vi "jitterPlot.vi"(8 "Y-jitter":dbl=0.03, 9 "X-jitter":dbl=0.03, 11 "PlotCluster":cluster{"X":dbl[], "Y":dbl[]}) -> (3 "JitteredPlotCluster":cluster{"X":dbl[], "Y":dbl[]})   [LabVIEW 2013]
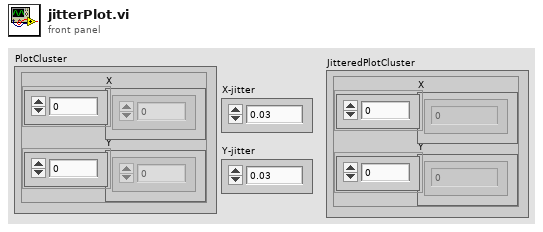
[diagram p1: front panel]
types:
  T1 = cluster{"jitteredArray":dbl[], "jitteredArray":dbl[]}
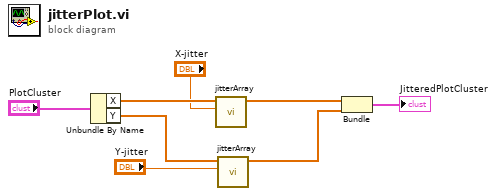
[diagram p0: block diagram]
diagram:
  n1 = Unbundle By Name("PlotCluster") -> ("X"=w6:dbl[], "Y"=w4:dbl[])
  n2 = call "jitterArray.vi"("Jitter"="X-jitter", "Array"=w6) -> ("jitteredArray"=w7:dbl[])  [unwired: 9 in]
  n3 = call "jitterArray.vi"("Jitter"="Y-jitter", "Array"=w4) -> ("jitteredArray"=w2:dbl[])  [unwired: 9 in]
  n4 = Bundle("jitteredArray"=w7, "jitteredArray"=w2) -> (→"JitteredPlotCluster":T1)  [unwired: 1 in]
